vi "gyro-frontend-server-18.vi"() -> ()   [LabVIEW 2020]
uses:
  icicle.ctl
  publisher action.ctl
panel:
  in  "Tab Control":enum32{"Page 1", "Page 2"}(tab)
  in  "wait (ms)":u32=20
  out "nanocal data":T1[](array[typedef])=[{"name"="frequency", "units"="Hz", "data"=59.21510317799475}, {"name"="Cs/T", "units"="J/K^2", "data"=1.24915044334812e-12}, {"name"="Ts", "units"="K", "data"=13.456821346295685}, {"name"="Cr/T", "units"="J/K^2", "data"=1.3468979938423544e-17}, {"name"="Tr", "units"="K", "data"=6.702259050679946}, {"name"="Ks", "units"="W/K", "data"=8.452345858606831e-09}, {"name"="Kr", "units"="W/K", "data"=1.5793868502253248e-14}, {"name"="Rs-therm", "units"="Ohm", "data"=4245.50086715559}, {"name"="Rr-therm", "units"="Ohm", "data"=5193.54439937376}]
  in  "Stop":bool
  # "gyro -- frontend server"
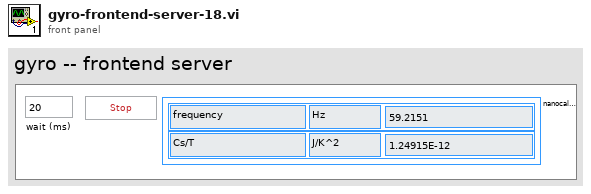
[diagram p1: front panel]
types:
  T1 = typedef "icicle.ctl" = cluster{"name":string, "units":string, "data":dbl}
  T2 = typedef "publisher action.ctl" = enum16{"set", "get", "init", "check"}
  T3 = typedef "pll talkback data type.ctl" = cluster{"freq (Hz)":dbl, "gamma (Hz)":dbl, "Voltage (V)":cdb, "overlimit ?":bool}
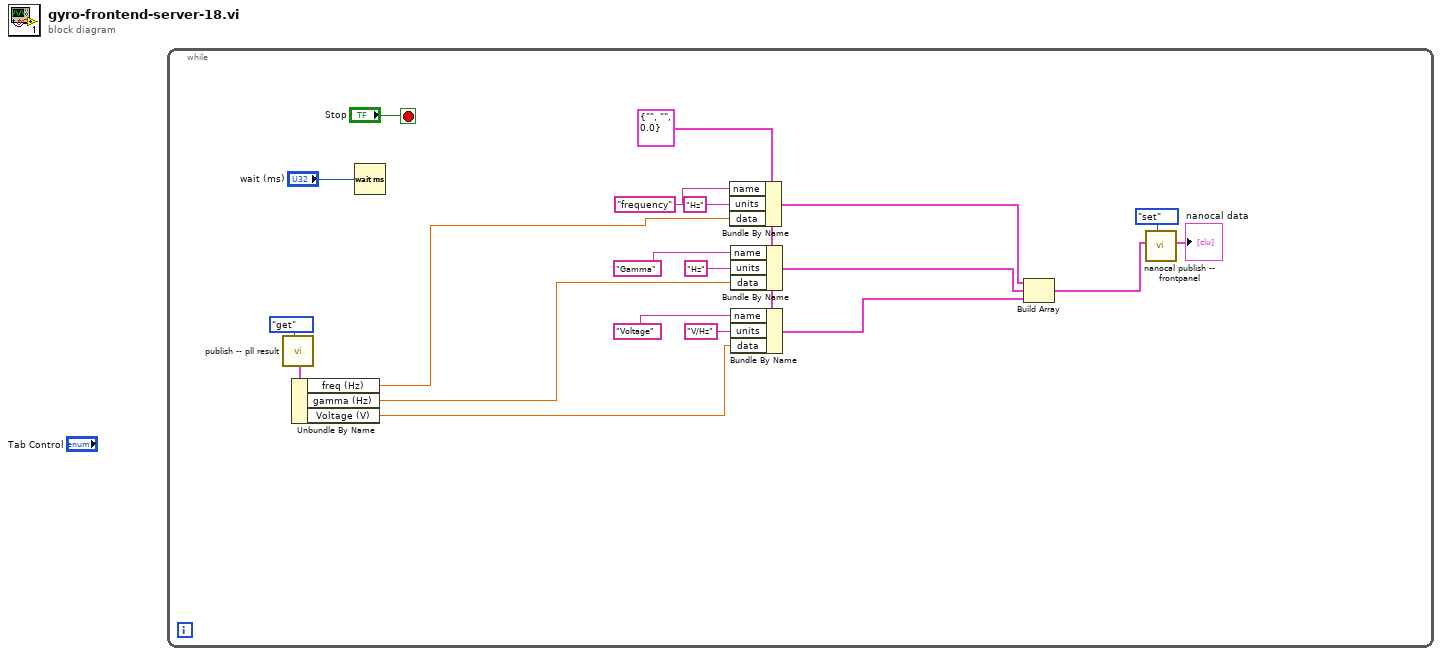
[diagram p0: block diagram]
diagram:
  n1 = while {
    stop <- "Stop" stop-if-true
    w10 = T1 {"name"="", "units"="", "data"=0.0} ("icicle")
    n2 = call "publish -- pll result.vi"("publisher action"=publisher_action."get") -> ("pll result OUT"=w8:T3)  [unwired: 10 in]
    n3 = Unbundle By Name(w8) -> ("freq (Hz)"=w7:dbl, "gamma (Hz)"=w6:dbl, "Voltage (V)"=w1:cdb)
    n4 = Wait (ms)(milliseconds to wait="wait (ms)") -> ()  [unwired: 1 out]
    n5 = Bundle By Name(cluster=w10, "name"="frequency", "units"="Hz", "data"=w7) -> (w5:T1)
    n6 = Bundle By Name(cluster=w10, "name"="Gamma", "units"="Hz", "data"=w6) -> (w4:T1)
    n7 = Bundle By Name(cluster=w10, "name"="Voltage", "units"="V/Hz", "data"=w1) -> (w3:T1)
    n8 = Build Array(w5, w4, w3) -> (w2:T1[])
    n9 = call "nanocal publish -- frontpanel.vi"("publisher action"=publisher_action."set", "nanocal data array IN"=w2) -> ("nanocal data array OUT"=→"nanocal data":T1[])  [unwired: 9 in]
  }
